vi "set_digital_output_value.vi"(0 "reference (in)":i32, 2 "digital_output_ch":T1, 3 "dig_out_value":bool, 5 "error in (no error)":errorcluster) -> (14 "reference (dup)":i32, 17 "response":string, 19 "error out":errorcluster)   [LabVIEW 2012]
doc: "This VI sets a the value to a single digital output channel of the attached device.\n\nProduced By:\n\nChristopher Lemieux\nKod Integrations, LLC\n4835 Marianne Drive\nMount Airy, MD 21771\nhttp://www.kodintegrations.com\nemail: clemieux@kodintegrations.com\nphone: (240) 687-1288"
uses:
  support/controls/digital_output_items.ctl
  main_functions/commands.ctl
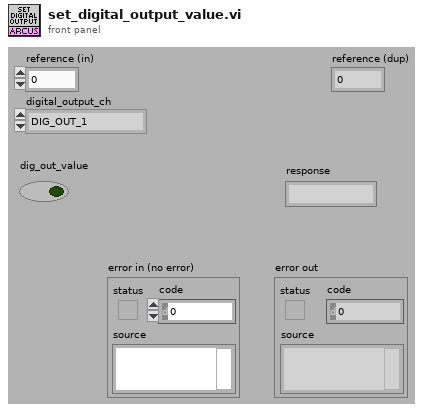
[diagram p1: front panel]
types:
  T1 = typedef "digital_output_items.ctl" = enum16{"DIG_OUT_1", "DIG_OUT_2"}
  T2 = typedef "commands.ctl" = enum16{"clear error", "constant jog(-)", "constant jog(+)", "get acceleration", "get actual current", "get device id", "get digital input status", "get digial inputs status", "get dig output status", "get digital outputs status", "get firmware ver", "get high speed", "get idle current", "get low speed", "get micro step", "get motor status", "get move mode", "get polarity", "get position", "get product id", "get power status", "get run current", "get status", "home(-)", "home(+)", "move to position", "power down", "power up", "set acceleration", "set device id", "set digital output", "set digital outputs", "set high speed", "set idle current", "set low speed", "set move mode absolute", "set move mode increment", "set polarity", "set position", "set run current", "stop immediate", "stop slow", "store to memory"}
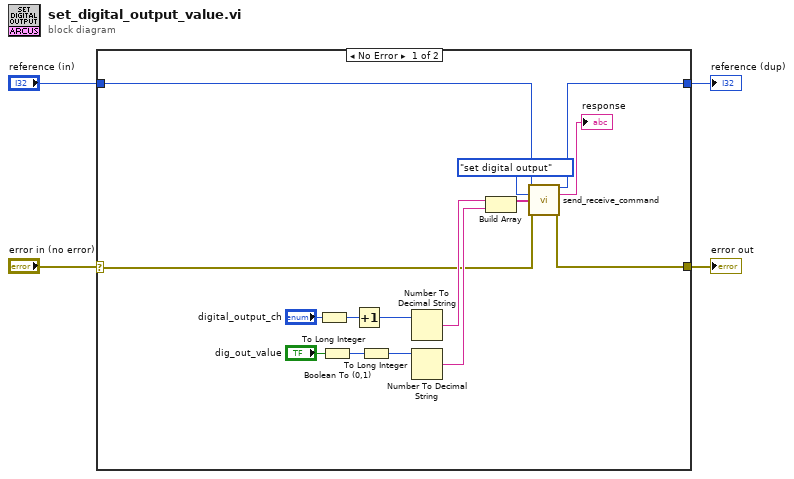
[diagram p0: block diagram]
diagram:
  n1 = case shown="No Error" "error in (no error)" {
    selector: "error in (no error)" -> [w11 w21]
    tunnel: [w19 w20] -> w4
    tunnel: [w17 w21] -> w3
    tunnel: "reference (in)" -> [w8 w20]
    frame No Error {
      n2 = To Long Integer(number="digital_output_ch") -> (32bit integer=w9:i32)
      n3 = Boolean To (0,1)(Boolean="dig_out_value") -> (0, 1=w12:i16)
      n4 = Increment(x=w9) -> (x+1=w5:i32)
      n5 = To Long Integer(number=w12) -> (32bit integer=w10:i32)
      n6 = Number To Decimal String(number=w5) -> (decimal integer string=w15:string)  [unwired: 1 in]
      n7 = Number To Decimal String(number=w10) -> (decimal integer string=w14:string)  [unwired: 1 in]
      n8 = Build Array(w15, w14) -> (w16:string[])
      n9 = call "send_receive_command.vi"("reference (in)"=w8, "command"=commands."set digital output", "params (opt)"=w16, "error in (no error)"=w11) -> ("reference (dup)"=w19:i32, "read_string"=→"response":string, "error out"=w17:errorcluster)  [unwired: 7 in, 2 out]
    }
    frame Error {
    }
  }
  "reference (dup)" <- w4
  "error out" <- w3
